vi "Convergence Status DAO.vi"(8 "error in (no error)":errorcluster, 9 "Convergence Status In":T3, 10 "LBCB Selected":T2, 11 "Actions":T1) -> (0 "error out":errorcluster, 3 "Convergence Status Out":T3)   [LabVIEW 2013]
uses:
  Mixed Mode Convergence Status.ctl
  Data Access Objects/Metadata/LBCB Number.ctl
  Data Access Objects/Metadata/DAO Actions.ctl
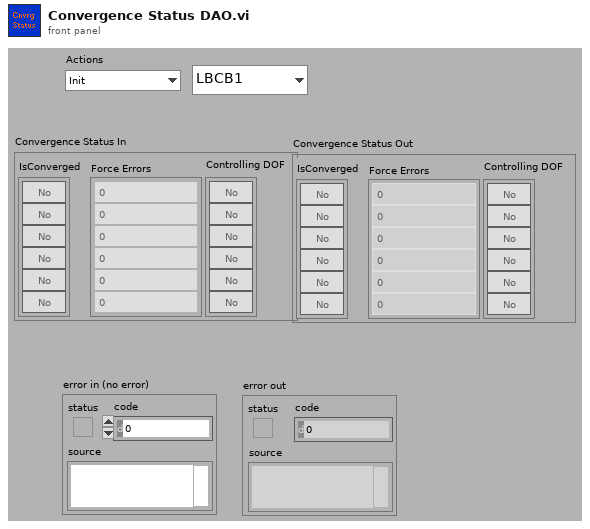
[diagram p1: front panel]
types:
  T1 = typedef "DAO Actions.ctl" = enum16{"Init", "Get", "Set"}
  T2 = typedef "LBCB Number.ctl" = enum16{"LBCB1", "LBCB2"}
  T3 = typedef "Mixed Mode Convergence Status.ctl" = cluster{"IsConverged":bool[], "Force Errors":dbl[], "Controlling DOF":bool[]}
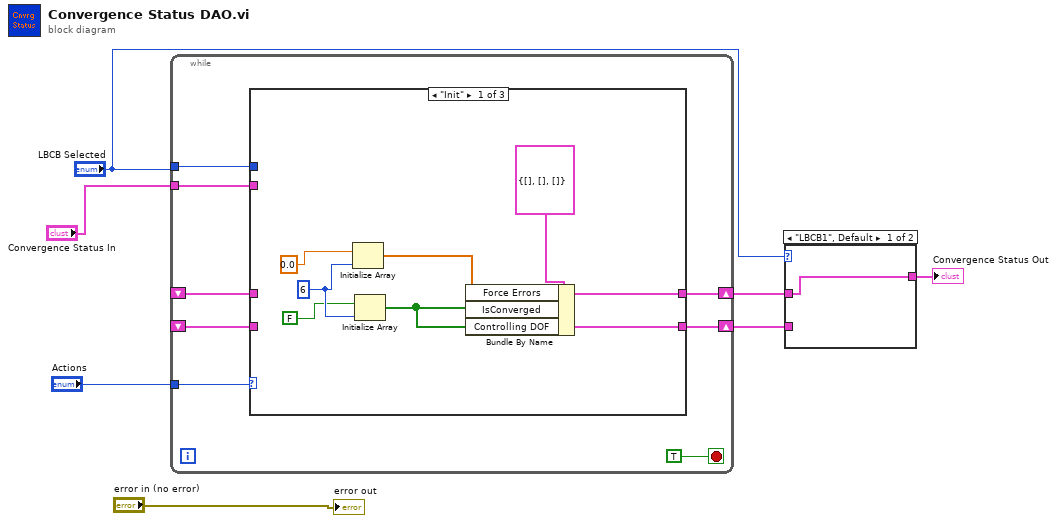
[diagram p0: block diagram]
diagram:
  n1 = while {
    tunnel: "Actions" -> [w14]
    tunnel: "LBCB Selected" -> [w13]
    tunnel: "Convergence Status In" -> [w12]
    shift-right: [w11] -> w4
    shift-left: _ -> [w9]
    shift-right: [w10] -> w3
    shift-left: _ -> [w8]
    stop <- TRUE stop-if-true
    n2 = case shown="\"Init\"" w14 {
      tunnel: w13 -> [_ w28 _]
      tunnel: w12 -> [_ w27 _]
      tunnel: [w18 w26 w33] -> w11
      tunnel: [w18 w25 w34] -> w10
      tunnel: w9 -> [_ w24 w33]
      tunnel: w8 -> [_ w23 w34]
      frame "Init" {
        w20 = 6 ("dimension size")
        n3 = Initialize Array(0.0, w20) -> (w17:dbl[])
        n4 = Initialize Array(FALSE, w20) -> (w16:bool[])
        n5 = Bundle By Name(cluster=T3 {"IsConverged"=[], "Force Errors"=[], "Controlling DOF"=[]} ("Convergence Status In"), "Force Errors"=w17, "IsConverged"=w16, "Controlling DOF"=w16) -> (w18:T3)
      }
      frame "Set" {
        n6 = case shown="\"LBCB2\"" w28 {
          tunnel: w27 -> [w30 w32]
          tunnel: [w29 w32] -> w26
          tunnel: [w30 w31] -> w25
          tunnel: w24 -> [w29 _]
          tunnel: w23 -> [_ w31]
          frame "LBCB1", Default {
          }
          frame "LBCB2" {
          }
        }
      }
      frame "Get", Default {
      }
    }
  }
  n7 = case shown="\"LBCB1\", Default" "LBCB Selected" {
    tunnel: w4 -> [_ w36]
    tunnel: w3 -> [w35 _]
    tunnel: [w35 w36] -> w2
    frame "LBCB1", Default {
    }
    frame "LBCB2" {
    }
  }
  "Convergence Status Out" <- w2
  "error out" <- "error in (no error)"
